vi "RealTimeAcq.vi"(4 "Frames/s":sgl=2.0, 5 "return to start":bool, 6 "Scan Axis":i8=3, 7 "Motion Board ID":T2=1 min=1 max=32 step=1, 8 "BKPT Shift":i32=75, 9 "stop out":bool) -> (0 "error out":errorcluster, 2 "Bd ID Out":T1)   [LabVIEW 2022 SP3]
uses:
  ScanningControl/Motion Controllers/-MotionRoutines/MotionGlobals.vi
  <instrlib>/Acqiris Dx/Acqiris Dx.lvlib
  <vilib>/Motion/FlexMotion/FunctionsVIs/Trajectory.llb/Load Acceleration/Deceleration.flx
  <vilib>/Motion/FlexMotion/CustomControls/CustomControls.llb/Axis To Control.flx
  <vilib>/Motion/FlexMotion/CustomControls/CustomControls.llb/Program.flx
  <instrlib>/Newport ESP301/Newport ESP301.lvlib
  <instrlib>/niScope/Acquire/Fetch/niScope Multi Fetch Binary 8.vi
  ScanningControl/-ScanSystem/DataHandling/ReverseDataI8.vi
  <vilib>/DAQmx/write.llb/DAQmx Write (Digital 1D Bool NChan 1Samp 1Line).vi
  <instrlib>/LeCroy Wave Series/LeCroy Wave Series.lvlib
  <vilib>/Motion/FlexMotion/FunctionsVIs/Trajectory.llb/Wait for Move Complete (8 axes).flx
panel:
  out "Frames":i32
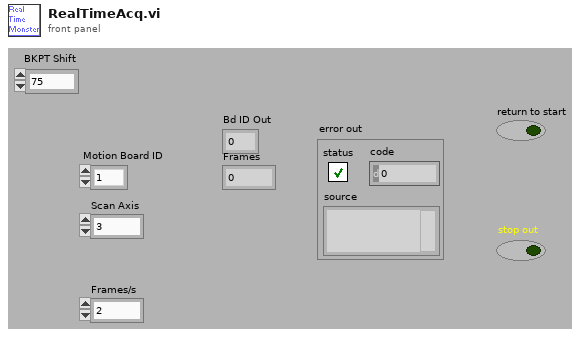
[diagram p1: front panel]
types:
  T1 = typedef "Bd Id Out" = u8
  T2 = typedef "Board Id" = u8
  T3 = cluster{"Time Step (ms)":i64, "Burst Ct":i8[], "Voltage Steps":sgl[], "Tabor Step Through?":bool}
  T4 = typedef "location.ctl" = enum16{"Automatic", "WCM Main", "Hawaii", "Columbia MM3000", "Columbia  NI System", "NYU", "RRI 2", "UHI Allen", "CUMC RT", "Chiba", "Stony Brook", "WCM Microscopy", "WCM Aeoretch", "WCM Optics Lab", "WCM Main 2Axis", "WCM Rotation", "WCM SAM SMAC", "SERI GP"}
  T5 = typedef "Program.flx" = u8
  T6 = cluster{"gain":dbl, bool, "Array":i16[][], "gain 2":dbl}
  T7 = typedef "Resource Out (Enum).flx" = u16
  T8 = typedef "Axis To Control.flx" = u16
  T9 = cluster{"returnedSamplesPerSeg":i32, "indexFirstPoint":i32, "sampTime":dbl, "vGain":dbl, "vOffset":dbl, "returnedSegments":i32, "nbrAvgWforms":i32, "actualTriggersInAcqLo":u32, "actualTriggersInAcqHi":u32, "reserved3":dbl, "actualDataSize":u32, "missingValue":dbl}
  T10 = cluster{"actualSamples":i32, "absoluteInitialX":dbl, "relativeInitialX":dbl, "xIncrement":dbl, "offset":dbl, "gain":dbl, "reserved1":dbl, "reserved2":dbl}[]
  T11 = cluster{"actualSamples":i32, "absoluteInitialX":dbl, "relativeInitialX":dbl, "xIncrement":dbl, "offset":dbl, "gain":dbl, "reserved1":dbl, "reserved2":dbl}
  T12 = cluster{"gain":dbl, bool, "Array":i16[][], "gain 2 Ch":dbl}
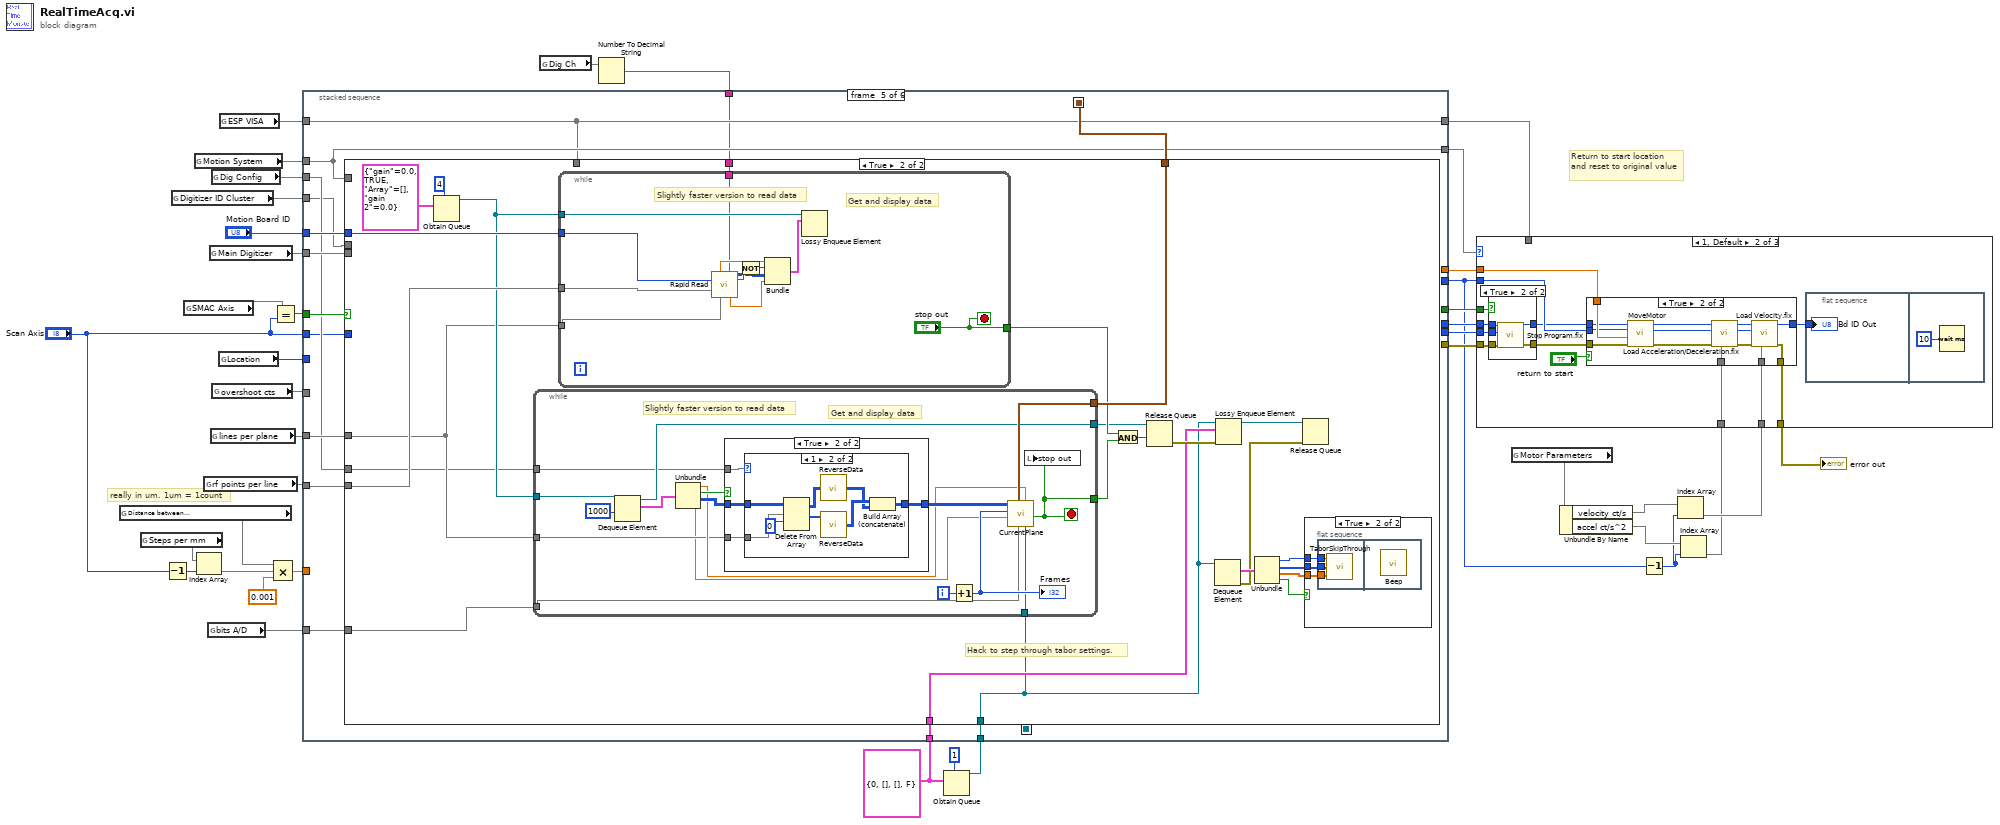
[diagram p0: block diagram]
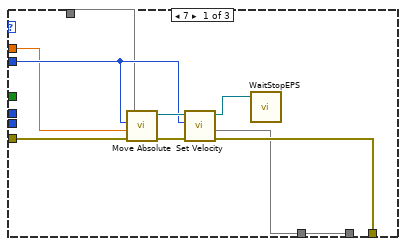
[diagram p2: hidden frame]
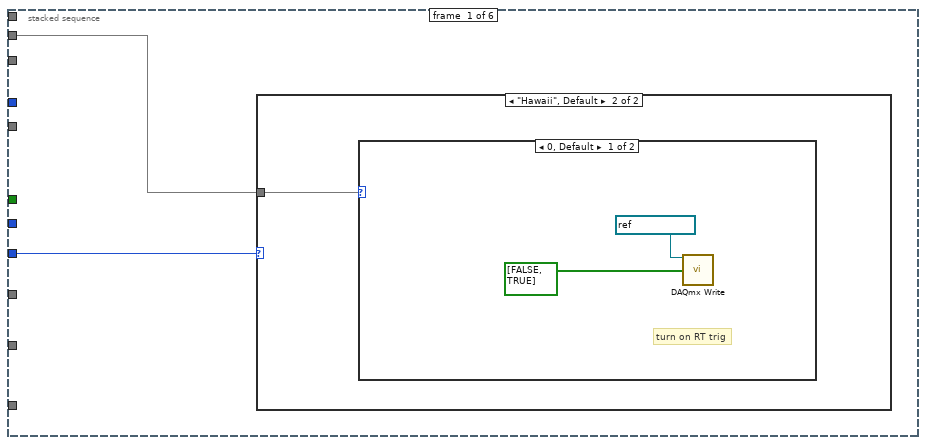
[diagram p6: hidden frame]
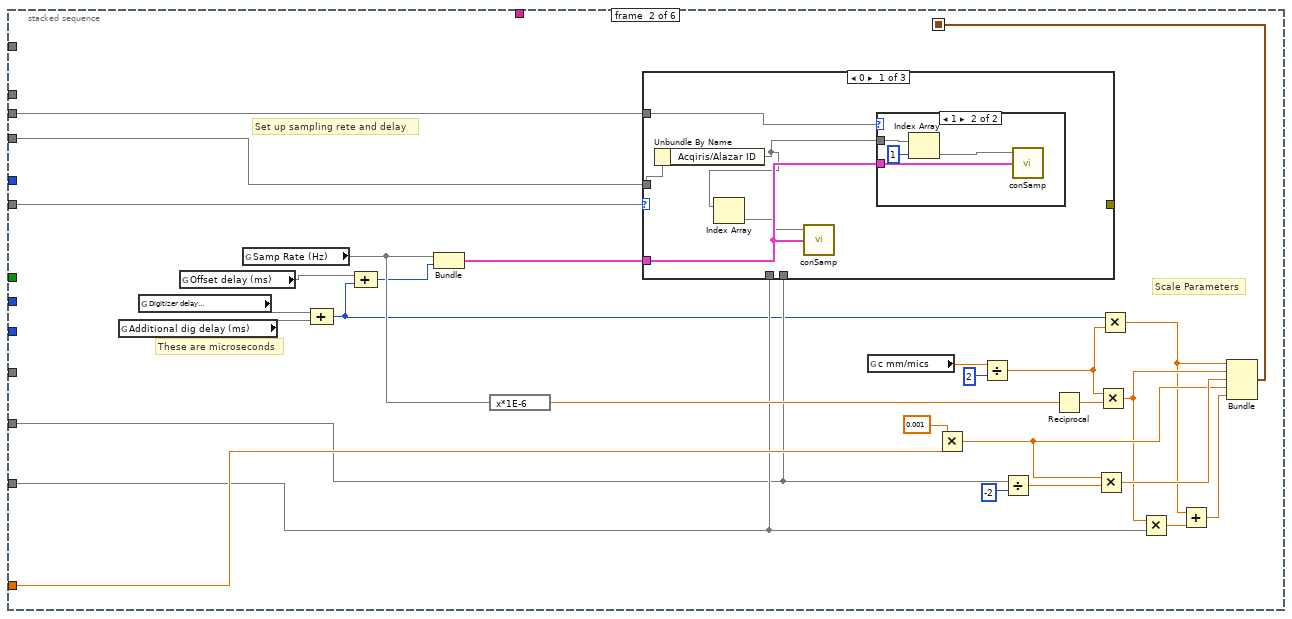
[diagram p9: hidden frame]
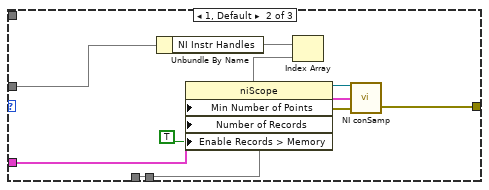
[diagram p11: hidden frame]
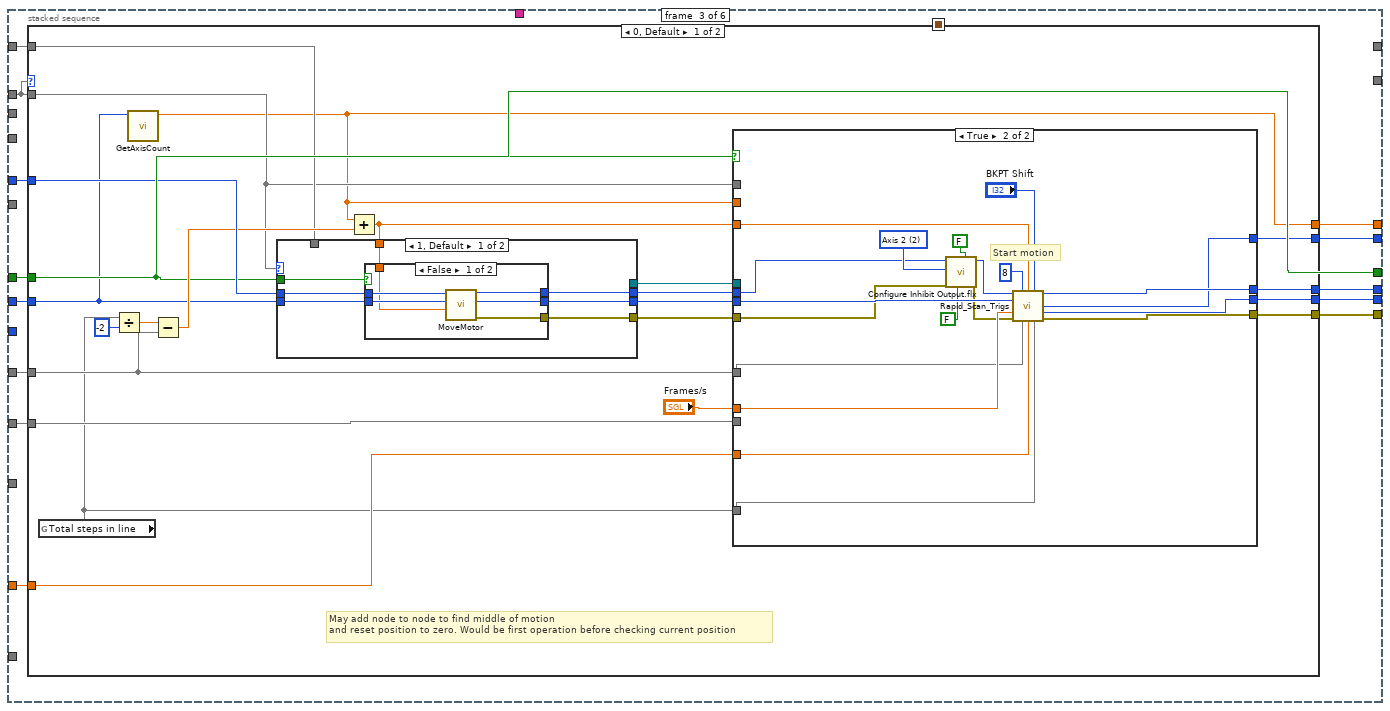
[diagram p13: hidden frame]
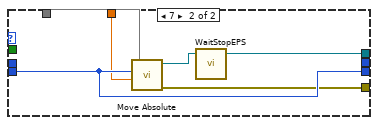
[diagram p15: hidden frame]
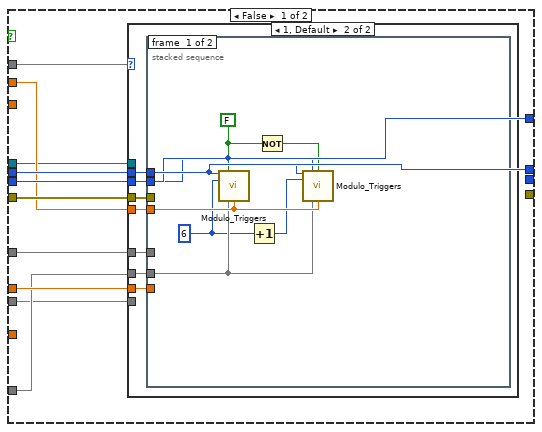
[diagram p16: hidden frame]
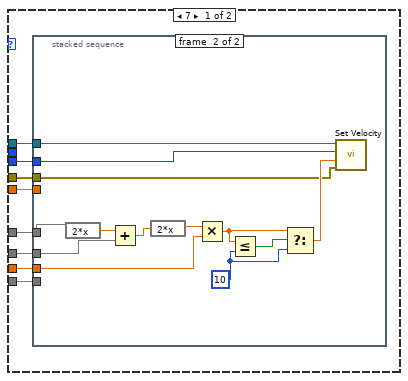
[diagram p17: hidden frame]
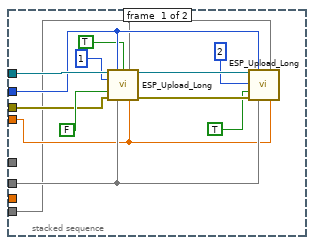
[diagram p18: hidden frame]
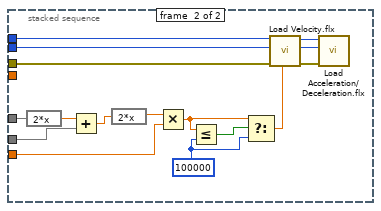
[diagram p19: hidden frame]
diagram:
  w11 = T3 {"Time Step (ms)"=0, "Burst Ct"=[], "Voltage Steps"=[], "Tabor Step Through?"=FALSE} ("Tabor")
  # "really in um. 1um = 1count"
  # "Return to start location and reset to original value"
  n1 = global read "MotionGlobals.vi" "Distance between\nscan lines (mm)"() -> (w29)
  n2 = global read "MotionGlobals.vi" "Steps per mm"() -> (w16)
  n3 = Decrement(x="Scan Axis") -> (x-1=w15:i8)
  n4 = global read "MotionGlobals.vi" "Digitizer ID Cluster"() -> (w9)
  n5 = global read "MotionGlobals.vi" "SMAC Axis"() -> (w13)
  n6 = global read "MotionGlobals.vi" "Motion System"() -> (w26)
  n7 = Index Array(array=w16, index=w15) -> (element=w14)
  n8 = global read "MotionGlobals.vi" "rf points per line"() -> (w39)
  n9 = global read "MotionGlobals.vi" "bits A/D"() -> (w17)
  n10 = global read "MotionGlobals.vi" "Main Digitizer"() -> (w27)
  n11 = global read "MotionGlobals.vi" "lines per plane"() -> (w40)
  n12 = global read "MotionGlobals.vi" "Dig Config"() -> (w20)
  n13 = global read "MotionGlobals.vi" "overshoot cts"() -> (w38)
  n14 = global read "MotionGlobals.vi" "Location"() -> (w21:T4)
  n15 = global read "MotionGlobals.vi" "ESP VISA"() -> (w25)
  n16 = Equal?(x=w13, y="Scan Axis") -> (x = y?=w31:bool)
  n17 = Compound Arithmetic op=MULTIPLY(w29, w14, 0.001) -> (w28:dbl)
  n18 = global read "MotionGlobals.vi" "Dig Ch"() -> (w19)
  n19 = Number To Decimal String(number=w19) -> (decimal integer string=w18:string)  [unwired: 1 in]
  n20 = Obtain Queue(max queue size (-1, unlimited)=1, element data type=w11) -> (queue out=w10:refnum<queue>)  [unwired: 3 in, 2 out]
  n21 = stacked-sequence {
    seq-local: [_ w63 _ _ _ _] -> [_ _ _ _ w286 _]
    seq-local: [_ _ _ w244 _ _] -> [_ _ _ _ _ w544]
    tunnel: w40 -> [_ w51 w98 _ w289 _]
    tunnel: [_ _ w105 _ _ _] -> w35
    tunnel: [_ _ w104 _ _ _] -> w37
    tunnel: w39 -> [_ w52 _ _ w288 _]
    tunnel: [_ _ w103 _ _ _] -> w36
    tunnel: [_ _ w94 _ _ _] -> w34
    tunnel: w38 -> [_ _ w101 _ _ _]
    tunnel: [_ _ w102 _ _ _] -> w1
    tunnel: "Motion Board ID" -> [_ _ w100 w245 w287 _]
    tunnel: [_ _ w95 _ _ _] -> w32
    tunnel: w31 -> [_ _ w95 _ w285 _]
    tunnel: "Scan Axis" -> [_ _ w96 w246 w278 _]
    tunnel: w28 -> [_ w56 w99 _ _ _]
    tunnel: w27 -> [_ w55 _ _ w284 _]
    tunnel: w26 -> [_ _ w93 w248 w283 _]
    tunnel: w25 -> [_ _ w97 _ w282 _]
    tunnel: [_ _ _ _ w283 _] -> w24
    tunnel: [_ _ _ _ w282 _] -> w23
    tunnel: w21 -> [w42 _ _ _ _ w547]
    tunnel: w20 -> [w41 w47 _ w247 w281 w545]
    tunnel: w18 -> [_ _ _ _ w280 _]
    tunnel: w17 -> [_ _ _ _ w279 _]
    tunnel: w11 -> [_ _ _ _ w277 _]
    tunnel: w10 -> [_ _ _ _ w276 _]
    tunnel: w9 -> [_ w46 _ _ w275 _]
    frame #0 {
      n22 = case shown="\"Hawaii\", Default" w42 {
        tunnel: w41 -> [_ w43]
        frame "UHI Allen", "CUMC RT" {
        }
        frame "Hawaii", Default {
          n23 = case shown="0, Default" w43 {
            frame 0, Default {
              # "turn on RT trig"
              n24 = call-poly <vilib>:"DAQmx Write.vi"("task/channels in"=refnum<k21> "DIO-L2 L3", "data"=bool[] [FALSE, TRUE]) -> ()  [unwired: 11 in, 3 out]
            }
            frame 44 {
            }
          }
        }
      }
    }
    frame #1 {
      # "Scale Parameters"
      # "Set up sampling rete and delay"
      # "These are microseconds"
      n25 = global read "MotionGlobals.vi" "Additional dig delay (ms)"() -> (w73)
      n26 = global read "MotionGlobals.vi" "Digitizer delay\n (ms)"() -> (w70)
      n27 = global read "MotionGlobals.vi" "Offset delay (ms)"() -> (w50)
      n28 = global read "MotionGlobals.vi" "Samp Rate (Hz)"() -> (w54)
      n29 = Compound Arithmetic op=ADD(w70, w73) -> (w49:i32)
      n30 = Compound Arithmetic op=ADD(w50, w49) -> (w48:i32)
      n31 = Bundle("Samp Rate (Hz)"=w54, w48) -> (w72:cluster{"Samp Rate (Hz)":void, i32})  [unwired: 1 out]
      n32 = expression code="x*1E-6"(w54) -> (w53:dbl)
      n33 = case shown="0" w55 {
        tunnel: w72 -> [w78 w88 _]
        tunnel: w46 -> [w76 w85 _]
        tunnel: w52 -> [_ w91 _]
        tunnel: w51 -> [_ w92 _]
        tunnel: [_ w87 _] -> _
        tunnel: w47 -> [w77 _ _]
        frame 0 {
          n34 = Unbundle By Name(w76) -> ("Acqiris/Alazar ID"=w75)
          n35 = Index Array(array=w75) -> (element=w74)  [unwired: 1 in]
          n36 = call "conSamp.vi"("Sampling"=w78, "InstrumentID"=w74) -> ()  [unwired: 1 in, 2 out]
          n37 = case shown="1" w77 {
            tunnel: w78 -> [_ w82]
            tunnel: w75 -> [_ w80]
            frame 0, Default {
            }
            frame 1 {
              n38 = Index Array(array=w80, index=1) -> (element=w79)
              n39 = call "conSamp.vi"("Sampling"=w82, "InstrumentID"=w79) -> ()  [unwired: 1 in, 2 out]
            }
          }
        }
        frame 1, Default {
          n40 = Unbundle By Name(w85) -> ("NI Instr Handles"=w84)
          n41 = Index Array(array=w84) -> (element=w83)  [unwired: 1 in]
          n42 = property class="niScope"(reference=w83, "Min Number of Points"=w91, "Number of Records"=w92, "Enable Records > Memory"=TRUE) -> (reference out=w90:refnum<k15>, error out=w89:errorcluster)  [unwired: 1 in]
          n43 = call "NI conSamp.vi"("error in"=w89, "Sampling"=w88, "InstrumentID"=w90) -> ("error out"=w87:errorcluster)  [unwired: 1 out]
        }
        frame 2 {
        }
      }
      n44 = global read "MotionGlobals.vi" "c mm/mics"() -> (w71:sgl)
      n45 = Multiply(x=0.001, y=w56) -> (x*y=w61:dbl)
      n46 = Divide(x=w71, y=2) -> (x/y=w64:sgl)
      n47 = Divide(x=w51, y=-2) -> (x/y=w66:dbl)
      n48 = Reciprocal(x=w53) -> (1/x=w69:dbl)
      n49 = Multiply(x=w61, y=w66) -> (x*y=w62:dbl)
      n50 = Multiply(x=w64, y=w69) -> (x*y=w60:dbl)
      n51 = Multiply(x=w49, y=w64) -> (x*y=w58:sgl)
      n52 = Multiply(x=w60, y=w52) -> (x*y=w59:dbl)
      n53 = Add(x=w58, y=w59) -> (x+y=w57:sgl)
      n54 = Bundle(w58, w60, w62, w61, w57) -> (w63:cluster{sgl, dbl, dbl, dbl, sgl})  [unwired: 1 out]
    }
    frame #2 {
      n55 = case shown="0, Default" w93 {
        tunnel: [w127 _] -> w105
        tunnel: [w126 _] -> w104
        tunnel: [w124 _] -> w103
        tunnel: [w123 _] -> w102
        tunnel: w101 -> [w121 _]
        tunnel: w100 -> [w117 _]
        tunnel: w99 -> [w116 _]
        tunnel: w98 -> [w114 _]
        tunnel: w97 -> [w113 _]
        tunnel: w96 -> [w107 _]
        tunnel: w95 -> [w110 _]
        tunnel: [w106 _] -> w94
        tunnel: w93 -> [w109 _]
        frame 0, Default {
          # "May add node to node to find middle of motion\nand reset position to zero. Would be first operation before checking current position"
          n56 = global read "MotionGlobals.vi" "Total steps in line"() -> (w108)
          n57 = Divide(x=w108, y=-2) -> (x/y=w122:dbl)
          n58 = call "GetAxisCount.vi"("Scan Axis"=w107) -> ("Counts"=w106:dbl)  [unwired: 10 in]
          n59 = Subtract(x=w122, y=w121) -> (x-y=w115:dbl)
          n60 = Add(x=w106, y=w115) -> (x+y=w111:dbl)
          n61 = case shown="1, Default" w109 {
            tunnel: [w133 _] -> w120
            tunnel: [w132 w149] -> w119
            tunnel: [w131 w146] -> w118
            tunnel: w117 -> [w135 _]
            tunnel: w107 -> [w134 w149]
            tunnel: w113 -> [_ w145]
            tunnel: [_ w147] -> w112
            tunnel: w111 -> [w130 w144]
            tunnel: w110 -> [w129 _]
            frame 1, Default {
              n62 = case shown="False" w129 {
                tunnel: w135 -> [w141 w143]
                tunnel: w134 -> [w140 w142]
                tunnel: [w139 w143] -> w133
                tunnel: [w138 w142] -> w132
                tunnel: [w137 _] -> w131
                tunnel: w130 -> [w136 _]
                frame False {
                  n63 = call "MoveMotor.vi"("Target Position (0)"=w136, "Axis or Vector Space"=w140, "Motion Bd ID"=w141) -> ("error out"=w137:errorcluster, "Resource Output"=w138:u16, "Bd ID Out"=w139:u8)  [unwired: 2 in, 4 out]
                }
                frame True {
                }
              }
            }
            frame 7 {
              n64 = call <instrlib>:"Move Absolute.vi"("Position (0 units)"=w144, "Axis (1)"=w149, "VISA resource name"=w145) -> ("error out"=w146:errorcluster, "VISA resource name out"=w148:refnum<visa-resource-name>)  [unwired: 3 in]
              n65 = call "WaitStopEPS.vi"("VISA resource name"=w148) -> ("VISA resource name out"=w147:refnum<visa-resource-name>)  [unwired: 2 in, 2 out]
            }
          }
          n66 = case shown="True" w110 {
            tunnel: "Frames/s" -> [w156 w243]
            tunnel: [_ w242] -> w127
            tunnel: [w159 w241] -> w126
            tunnel: [_ w240] -> w124
            tunnel: [w158 w239] -> w123
            tunnel: w108 -> [w153 w238]
            tunnel: w116 -> [_ w237]
            tunnel: w121 -> [w157 w236]
            tunnel: w120 -> [w159 w226]
            tunnel: w119 -> [w158 w235]
            tunnel: w118 -> [w155 w225]
            tunnel: w111 -> [_ w234]
            tunnel: w106 -> [w154 _]
            tunnel: w114 -> [w152 _]
            tunnel: w109 -> [w151 _]
            tunnel: w112 -> [w150 _]
            frame False {
              n67 = case shown="1, Default" w151 {
                tunnel: w153 -> [w167 w200]
                tunnel: w159 -> [_ w199]
                tunnel: w158 -> [w162 w198]
                tunnel: w157 -> [w164 w197]
                tunnel: w156 -> [w163 w196]
                tunnel: w155 -> [w160 w195]
                tunnel: w154 -> [w165 w194]
                tunnel: w152 -> [w166 _]
                tunnel: w150 -> [w161 _]
                frame 7 {
                  n68 = stacked-sequence {
                    tunnel: w167 -> [w172 w186]
                    tunnel: w166 -> [w169 _]
                    tunnel: w165 -> [w171 _]
                    tunnel: w164 -> [_ w187]
                    tunnel: w163 -> [_ w185]
                    tunnel: w162 -> [w170 w183]
                    tunnel: w161 -> [w180 w182]
                    tunnel: w160 -> [w175 w181]
                    frame #0 {
                      n69 = call "ESP_Upload_Long.vi"("Motion Settings In"=w180, "Axis"=w170, "Purge?"=TRUE, "lines per scan"=w169, "Program#"=1, "Reverse ?"=FALSE, "error in"=w175, 12:w172, "Offset"=w171) -> ("VISA resource name out"=w179:refnum<visa-resource-name>, "error out"=w174:errorcluster)  [unwired: 5 in]
                      n70 = call "ESP_Upload_Long.vi"("Motion Settings In"=w179, "Axis"=w170, "lines per scan"=w169, "Program#"=2, "Reverse ?"=TRUE, "error in"=w174, 12:w172, "Offset"=w171) -> ()  [unwired: 6 in, 2 out]
                    }
                    frame #1 {
                      w192 = 10
                      n71 = expression code="2*x"(w187) -> (w190:dbl)
                      n72 = Add(x=w190, y=w186) -> (x+y=w188:dbl)
                      n73 = expression code="2*x"(w188) -> (w189:dbl)
                      n74 = Multiply(x=w189, y=w185) -> (x*y=w193:sgl)
                      n75 = Less Or Equal?(x=w193, y=w192) -> (x <= y?=w191:bool)
                      n76 = Select(t=w193, s=w191, f=w192) -> (s? t:f=w184:sgl)
                      n77 = call <instrlib>:"Set Velocity.vi"("error in (no error)"=w181, "Velocity (units/s)"=w184, "Axis (1)"=w183, "VISA resource name"=w182) -> ()  [unwired: 2 in, 2 out]
                    }
                  }
                }
                frame 1, Default {
                  n78 = stacked-sequence {
                    tunnel: w194 -> [w208 _]
                    tunnel: w200 -> [w207 w221]
                    tunnel: w199 -> [w203 w217]
                    tunnel: w198 -> [w202 w216]
                    tunnel: w197 -> [_ w214]
                    tunnel: w196 -> [_ w212]
                    tunnel: w195 -> [_ w218]
                    frame #0 {
                      w201 = T5 6 ("Program (1)")
                      w206 = FALSE
                      n79 = call "Modulo_Triggers.vi"("Motion Settings In"=w203, "Axis"=w202, "Reverse ?"=w206, "Program (1)"=w201, 12:w207, "Offset"=w208) -> ()  [unwired: 2 in, 8 out]
                      n80 = Increment(x=w201) -> (x+1=w204:T5)
                      n81 = Not(x=w206) -> (.not. x?=w205:bool)
                      n82 = call "Modulo_Triggers.vi"("Motion Settings In"=w203, "Axis"=w202, "Reverse ?"=w205, "Program (1)"=w204, 12:w207, "Offset"=w208) -> ()  [unwired: 2 in, 8 out]
                    }
                    frame #1 {
                      w223 = 100000
                      n83 = expression code="2*x"(w214) -> (w213:dbl)
                      n84 = Add(x=w213, y=w221) -> (x+y=w210:dbl)
                      n85 = expression code="2*x"(w210) -> (w211:dbl)
                      n86 = Multiply(x=w211, y=w212) -> (x*y=w224:sgl)
                      n87 = Less Or Equal?(x=w224, y=w223) -> (x <= y?=w222:bool)
                      n88 = Select(t=w224, s=w222, f=w223) -> (s? t:f=w209:sgl)
                      n89 = call <vilib>:"Load Velocity.flx"("Velocity (10000)"=w209, "error in (no error)"=w218, "Axis or Vector Space"=w216, "Board ID"=w217) -> ("error out"=w219:errorcluster, "Resource Output"=w215:T7, "Bd ID Out"=w220:T1)  [unwired: 3 out]
                      n90 = call "Load Acceleration/Deceleration.flx"("error in (no error)"=w219, "Axis or Vector Space"=w215, "Board ID"=w220) -> ()  [unwired: 2 in, 5 out]
                    }
                  }
                }
              }
            }
            frame True {
              w229 = T8 2 items=["Axis 1"=1, "Axis 2"=2, "Axis 3"=3, "Axis 4"=4, "Axis 5"=5, "Axis 6"=6, "Axis 7"=7, "Axis 8"=8] ("Axis")
              # "Start motion"
              n91 = call <vilib>:"Configure Inhibit Output.flx"("Enable"=FALSE, "Polarity (Active Low)"=FALSE, "error in (no error)"=w225, "Axis"=w229, "Board ID"=w226) -> ("error out"=w232:errorcluster, "Bd ID Out"=w233:T1)  [unwired: 1 in, 4 out]
              n92 = call "Rapid_Scan_Trigs.vi"("Board ID"=w233, "Program (1)"=T5 8, "Start Position"=w234, "BKPT Shift"="BKPT Shift", "Scan Axis"=w235, "# frames/ s"=w243, "error in (no error)"=w232, "overshoot"=w236, "step interval"=w237, "Total Steps (one way)"=w238) -> ("Bd ID Out"=w241:u8, "Axis Resource out"=w239:u16, "Program ID"=w240:u8, "error out"=w242:errorcluster)  [unwired: 1 in, 1 out]
            }
          }
        }
        frame 8 {
        }
      }
    }
    frame #3 {
      n93 = case shown="4" w247 {
        tunnel: [_ w257] -> w244
        tunnel: w246 -> [_ w260]
        tunnel: w245 -> [_ w253]
        frame 0, Default {
        }
        frame 4 {
          n94 = global read "MotionGlobals.vi" "Switch T/R"() -> (w261)
          n95 = Decrement(x=w261) -> (x-1=w252:dbl)
          n96 = Replace Array Subset(array=bool[] [FALSE, FALSE, FALSE, FALSE, FALSE] ("XMIT"), new element=TRUE ("new element/subarray"), index=w252) -> (w249:bool[])
          n97 = call "5ChPulserTrigsNew.vi"("Motion Settings"=w253, "XMIT"=w249, "Axis"=w260) -> ("5CH Pulser Tasks"=w259:refnum<k21>[])  [unwired: 6 in, 1 out]
          n98 = for {
            tunnel: w259 -> [w273] mode=indexing
            tunnel: [w272] -> w257 mode=indexing
            tunnel: [w271] -> w256
            n99 = call <vilib>:"DAQmx Start Task.vi"("task/channels in"=w273) -> ("task out"=w272:refnum<k21>, "error out"=w271:errorcluster)  [unwired: 1 in, 12 out]
          }
          n100 = for {
            tunnel: bool[][] [[TRUE], [FALSE]] ("data") -> [w265] mode=indexing
            tunnel: w256 -> [_]
            tunnel: [w264] -> w254
            n101 = flat-sequence {
              tunnel: w265 -> [w268]
              tunnel: [w268] -> w266
              tunnel: w266 -> [w270]
              tunnel: [w269] -> w264
              frame #0 {
                n102 = Wait (ms)(milliseconds to wait=u32 25) -> ()  [unwired: 1 out]
              }
              frame #1 {
                n103 = call "DAQ Assistant"("data"=w270) -> ("error out"=w269:errorcluster)  [unwired: 17 in, 1 out]
              }
            }
          }
          n104 = for {
            N: 3 -> [_]
            tunnel: w253 -> [w263]
            tunnel: w254 -> [w262]
            n105 = call "ForceBreakPt.vi"("error in"=w262, "Bd ID in"=w263) -> ()  [unwired: 2 out]
          }
        }
      }
      n106 = case shown="0, Default" w248 {
        tunnel: w245 -> [w274 _]
        frame 0, Default {
          n107 = call "CheckLimStat.vi"("Motion Board ID"=w274) -> ()
        }
        frame 1, 7, 8 {
        }
      }
    }
    frame #4 {
      n108 = case shown="True" w285 {
        tunnel: w289 -> [w303 w476]
        tunnel: w288 -> [w304 w493]
        tunnel: w287 -> [w301 w492]
        tunnel: w286 -> [w300 w490]
        tunnel: w284 -> [w299 _]
        tunnel: w283 -> [w298 _]
        tunnel: w282 -> [w297 _]
        tunnel: w281 -> [_ w475]
        tunnel: w280 -> [w296 w473]
        tunnel: w279 -> [w295 w472]
        tunnel: w278 -> [w293 _]
        tunnel: w277 -> [_ w471]
        tunnel: w276 -> [w292 w470]
        tunnel: w275 -> [w290 _]
        frame False {
          n109 = global read "MotionGlobals.vi" "DigTimeOut"() -> (w294)
          n110 = while {
            tunnel: w304 -> [w332]
            tunnel: w303 -> [w323]
            shift-right: [w331] -> _
            shift-left: TRUE -> [w316]
            tunnel: w301 -> [w330]
            tunnel: w300 -> [w326]
            tunnel: w299 -> [w324]
            tunnel: w298 -> [w317]
            tunnel: w297 -> [w318]
            tunnel: w296 -> [w311]
            tunnel: w295 -> [w309]
            tunnel: w294 -> [w308]
            tunnel: w293 -> [w307]
            tunnel: w292 -> [w306]
            tunnel: [w306] -> w291
            tunnel: w290 -> [w305]
            i -> [w325]
            stop <- w329 stop-if-true
            # "Display data"
            # "Get data"
            # "This is slower version for heavier mass motors. Scan stop, read data, scan etc"
            n111 = Select(t="1", s=w316, f="2") -> (s? t:f=w313:string)
            n112 = Select(t=T5 6 ("Program (1)"), s=w316, f=T5 7 ("Program (1)")) -> (s? t:f=w321:T5)
            n113 = case shown="1, Default" w324 {
              tunnel: w332 -> [w352 w397 _]
              tunnel: w323 -> [w351 w392 w431]
              tunnel: w330 -> [w364 w410 w421]
              tunnel: [w363 w409 w445] -> w328
              tunnel: w321 -> [w359 w408 w444]
              tunnel: [w345 w402 w427] -> w310
              tunnel: w305 -> [w338 w385 w419]
              tunnel: w316 -> [w348 w399 w426]
              tunnel: [w349 w400 w428] -> w322
              tunnel: w317 -> [w343 _ w439]
              tunnel: w318 -> [w347 _ w442]
              tunnel: w313 -> [w346 _ w441]
              tunnel: [w341 w389 w425] -> w312
              tunnel: w311 -> [_ w398 _]
              tunnel: w308 -> [w340 w386 w430]
              tunnel: w307 -> [_ _ w420]
              frame 0 {
                n114 = Unbundle By Name(w338) -> ("Acqiris/Alazar ID"=w337)
                n115 = Index Array(array=w337) -> (element=w336)  [unwired: 1 in]
                n116 = call <instrlib>:"Configure Memory Settings.vi"("Number of Samples (1000)"=w352, "Number of Segments (1)"=w351, "Instrument ID"=w336) -> ("error out"=w362:errorcluster, "dup Instrument ID"=w360:u32)  [unwired: 1 in, 2 out]
                n117 = call <instrlib>:"Start Acquisition.vi"("error in (no error)"=w362, "Instrument ID"=w360) -> ("error out"=w358:errorcluster, "dup Instrument ID"=w361:u32)  [unwired: 2 in]
                n118 = stacked-sequence {
                  tunnel: w358 -> [w382]
                  tunnel: [w382] -> w357
                  frame #0 {
                    n119 = Wait (ms)(milliseconds to wait=20) -> ()  [unwired: 1 out]
                  }
                }
                n120 = case shown="7" w343 {
                  tunnel: w364 -> [w370 _]
                  tunnel: [w369 _] -> w363
                  tunnel: w359 -> [w368 _]
                  tunnel: w357 -> [w367 w375]
                  tunnel: [w366 w372] -> w356
                  tunnel: w347 -> [_ w374]
                  tunnel: w346 -> [_ w373]
                  tunnel: [_ w371] -> w344
                  frame 0, Default {
                    n121 = call <vilib>:"Run Program.flx"("error in (no error)"=w367, "Program (1)"=w368, "Board ID"=w370) -> ("error out"=w366:errorcluster, "Bd ID Out"=w369:T1)  [unwired: 4 out]
                  }
                  frame 7 {
                    n122 = call <instrlib>:"Execute Program.vi"("error in (no error)"=w375, "Program Name"=w373, "VISA resource name"=w374) -> ("error out"=w372:errorcluster, "VISA resource name out"=w371:refnum<visa-resource-name>)  [unwired: 3 in]
                  }
                }
                n123 = expression code="x*1000"(w340) -> (w339:dbl)
                n124 = stacked-sequence {
                  tunnel: w356 -> [w379]
                  tunnel: [w379] -> w355
                  frame #0 {
                    n125 = Wait (ms)(milliseconds to wait=20) -> ()  [unwired: 1 out]
                  }
                }
                n126 = call "WaitForSegs.vi"("Acqiris ID"=w361, "lines per plane"=w351, "error in"=w355, "Timeout"=w339) -> ("dup Instrument ID"=w354:u32, "error out"=w353:errorcluster)  [unwired: 2 out]
                n127 = call "GetWaveform.vi"("Acq ID Out"=w354, "Num Samps"=w352, "Num Segs"=w351, "error in"=w353) -> ("Acquired Waveform16 bit"=w350:i16[][], "dataDesc"=w342:T9, "error out"=w345:errorcluster)  [unwired: 2 in, 7 out]
                n128 = case shown="True" w348 {
                  tunnel: w350 -> [w376 w378]
                  tunnel: [w376 w377] -> w349
                  frame False {
                  }
                  frame True {
                    n129 = call "ReverseData.vi"("Array in"=w378) -> ("Array out"=w377:i16[][])
                  }
                }
                n130 = Unbundle By Name(w342) -> ("vGain"=w341:dbl)
                n131 = case shown="7" w343 {
                  tunnel: w344 -> [_ w365]
                  frame 0, Default {
                  }
                  frame 7 {
                    n132 = call "WaitStopEPS.vi"("VISA resource name"=w365) -> ()  [unwired: 2 in, 3 out]
                  }
                }
              }
              frame 1, Default {
                n133 = Unbundle By Name(w385) -> ("NI Instr Handles"=w384)
                n134 = Index Array(array=w384) -> (element=w383)  [unwired: 1 in]
                n135 = property class="niScope"(reference=w383, "Number of Records"=w392, "Min Number of Points"=w397) -> (reference out=w404:refnum<k15>, error out=w403:errorcluster)  [unwired: 1 in]
                n136 = call <instrlib>:"niScope Initiate Acquisition.vi"("instrument handle"=w404, "error in"=w403) -> ("instrument handle out"=w396:refnum<k15>, "error out"=w407:errorcluster)  [unwired: 1 in, 11 out]
                n137 = stacked-sequence {
                  tunnel: w407 -> [w417]
                  tunnel: [w417] -> w406
                  frame #0 {
                    n138 = Wait (ms)(milliseconds to wait=u32 5) -> ()  [unwired: 1 out]
                  }
                }
                n139 = call <vilib>:"Run Program.flx"("error in (no error)"=w406, "Program (1)"=w408, "Board ID"=w410) -> ("error out"=w405:errorcluster, "Bd ID Out"=w409:T1)  [unwired: 4 out]
                n140 = stacked-sequence {
                  tunnel: w405 -> [w414]
                  tunnel: [w414] -> w394
                  frame #0 {
                    n141 = Wait (ms)(milliseconds to wait=u32 20) -> ()  [unwired: 1 out]
                  }
                }
                n142 = property class="niScope"(reference=w396, error in=w394, "Fetch Record Number"=0, "Fetch Number of Records"=-1) -> (reference out=w395:refnum<k15>, error out=w393:errorcluster)
                n143 = call-poly <instrlib>:"niScope Fetch (poly).vi"("timeout"=w386, "error in"=w393, "numSamples"=w397, "channels"=w398, "instrument handle"=w395) -> ("error out"=w402:errorcluster, "wfm"=w401:i8[][], "wfm info"=w391:T10)  [unwired: 4 out]
                n144 = case shown="True" w399 {
                  tunnel: w401 -> [w411 w413]
                  tunnel: [w411 w412] -> w400
                  frame False {
                  }
                  frame True {
                    n145 = call-poly "ReversePoly.vi"("Array in"=w413) -> ("Array out"=w412:i8[][])
                  }
                }
                n146 = Index Array(array=w391) -> (element=w390:T11)  [unwired: 1 in]
                n147 = Unbundle By Name(w390) -> ("gain"=w389:dbl)
              }
              frame 2 {
                w438 = FALSE ("Continuous Acquisition Mode (T: On)")
                w436 = u16 2 items=["RealTime", "RIS", "Sequence", "Roll", "WaveStream"] ("Sample Mode (0: RealTime)")
                n148 = Unbundle By Name(w419) -> ("LeCroy VISA"=w418)
                n149 = call <instrlib>:"Configure Continuous Acquisition.vi"("Auto Trigger Enabled (T: Normal)"=w438, "Continuous Acquisition Mode (T: On)"=w438, "VISA resource name"=w418) -> ("error out"=w435:errorcluster, "VISA resource name out"=w437:refnum<visa-resource-name>)  [unwired: 7 in]
                n150 = call <instrlib>:"Configure Sample Mode.vi"("error in (no error)"=w435, "Number of Segments (2)"=w431, "Sample Mode (0: RealTime)"=w436, "VISA resource name"=w437) -> ("error out"=w434:errorcluster, "VISA resource name out"=w432:refnum<visa-resource-name>)  [unwired: 6 in]
                n151 = call <instrlib>:"Initiate.vi"("error in (no error)"=w434, "VISA resource name"=w432) -> ("error out"=w433:errorcluster)  [unwired: 8 in, 1 out]
                n152 = case shown="0, Default" w439 {
                  tunnel: w421 -> [w451 _]
                  tunnel: [w450 _] -> w445
                  tunnel: w444 -> [w449 _]
                  tunnel: w433 -> [w448 w456]
                  tunnel: [w447 w453] -> w443
                  tunnel: w442 -> [_ w455]
                  tunnel: w441 -> [_ w454]
                  tunnel: [_ w452] -> w440
                  frame 0, Default {
                    n153 = call <vilib>:"Run Program.flx"("error in (no error)"=w448, "Program (1)"=w449, "Board ID"=w451) -> ("error out"=w447:errorcluster, "Bd ID Out"=w450:T1)  [unwired: 4 out]
                  }
                  frame 7 {
                    n154 = call <instrlib>:"Execute Program.vi"("error in (no error)"=w456, "Program Name"=w454, "VISA resource name"=w455) -> ("error out"=w453:errorcluster, "VISA resource name out"=w452:refnum<visa-resource-name>)  [unwired: 3 in]
                  }
                }
                n155 = expression code="x*1000"(w430) -> (w422:dbl)
                n156 = stacked-sequence {
                  tunnel: w443 -> [w457]
                  tunnel: [w457] -> w423
                  frame #0 {
                    n157 = Wait (ms)(milliseconds to wait=40) -> ()  [unwired: 1 out]
                  }
                }
                n158 = call-poly <vilib>:"Wait for Move Complete.flx"("Timeout (10000 ms)"=w422, "error in (no error)"=w423, "Axis or Vector Space"=w420, "Board ID"=w421) -> ("error out"=w424:errorcluster)  [unwired: 4 in, 3 out]
                n159 = call "GetAcqSeqLeCroy.vi"("errorin"=w424, "save?"=FALSE, "Reverse?"=w426) -> ("Raw VGain (scale)"=w425:dbl, "Data Array"=w428:i16[][], "error out"=w427:errorcluster)  [unwired: 18 in, 4 out]
                n160 = case shown="7" w439 {
                  tunnel: w440 -> [_ w446]
                  frame 0, Default {
                  }
                  frame 7 {
                    n161 = call "WaitStopEPS.vi"("VISA resource name"=w446) -> ()  [unwired: 2 in, 3 out]
                  }
                }
              }
            }
            n162 = case shown="No Error" w310 {
              selector: w310 -> [w463 w468]
              tunnel: [w464 w468] -> w327
              tunnel: [w467 TRUE] -> w329
              tunnel: w326 -> [w466 _]
              tunnel: w325 -> [w465 _]
              tunnel: w322 -> [w462 _]
              tunnel: w312 -> [w461 _]
              tunnel: w309 -> [w460 _]
              tunnel: w306 -> [w459 _]
              frame No Error {
                n163 = call "CurrentPlane.vi"("queue In"=w459, "gain"=w461, "bits A/D"=w460, "Axis Vals"=w466, "error in"=w463, "Frame"=w465, "Data"=w462) -> ("error out"=w464:errorcluster, "stop out"=w467:bool)  [unwired: 3 in]
              }
              frame Error {
              }
            }
            n164 = local write "Frames"(w325) -> ()
            n165 = case shown="1, Default" w317 {
              tunnel: w328 -> [_ w335]
              tunnel: w327 -> [_ w334]
              tunnel: w321 -> [_ w333]
              frame 7 {
              }
              frame 1, Default {
                n166 = call <vilib>:"Stop Program.flx"("error in (no error)"=w334, "Program (1)"=w333, "Board ID"=w335) -> ()  [unwired: 6 out]
              }
            }
            n167 = Not(x=w316) -> (.not. x?=w331:bool)
          }
          n168 = Release Queue(queue=w291) -> ()  [unwired: 2 in, 3 out]
        }
        frame True {
          # "Hack to step through tabor settings."
          n169 = Obtain Queue(max queue size (-1, unlimited)=4, element data type=T6 {"gain"=0.0, TRUE, "Array"=[], "gain 2"=0.0}) -> (queue out=w489:refnum<queue>)  [unwired: 2 in, 3 out]
          n170 = while {
            tunnel: w490 -> [w515]
            tunnel: w489 -> [w508]
            tunnel: [w511] -> w487
            tunnel: [w513] -> w486
            tunnel: w470 -> [w504]
            tunnel: w475 -> [w503]
            tunnel: w476 -> [w502]
            tunnel: w472 -> [w500]
            i -> [w516]
            stop <- w511 stop-if-true
            # "Slightly faster version to read data"
            # "Get and display data"
            n171 = Dequeue Element(queue=w508, timeout in ms (-1)=1000) -> (queue out=w513:refnum<queue>, element=w510:T6)  [unwired: 1 in, 2 out]
            n172 = Unbundle(w510) -> ("gain"=w505:dbl, w506:bool, "Array"=w507:i16[][], "gain 2"=w501:dbl)
            n173 = case shown="True" w506 {
              tunnel: w507 -> [w517 w521]
              tunnel: [w517 w520] -> w509
              tunnel: w503 -> [_ w519]
              tunnel: w502 -> [_ w518]
              frame False {
              }
              frame True {
                n174 = case shown="1" w519 {
                  tunnel: w521 -> [w523 w531]
                  tunnel: [w522 w525] -> w520
                  tunnel: w518 -> [_ w530]
                  frame 0, Default {
                    n175 = call "ReverseData.vi"("Array in"=w523) -> ("Array out"=w522:i16[][])
                  }
                  frame 1 {
                    n176 = Delete From Array(array=w531, length=w530, index (row)=0 ("disabled index (col)")) -> (deleted portion=w528:i16[], array with subset deleted=w529:i16[][])  [unwired: 1 in]
                    n177 = call "ReverseData.vi"("Array in"=w529) -> ("Array out"=w526:i16[][])
                    n178 = call "ReverseData.vi"("Array in"=w528) -> ("Array out"=w527:i16[][])
                    n179 = Build Array (concatenate)(w527, w526) -> (w525:i16[][])
                  }
                }
              }
            }
            n180 = Increment(x=w516) -> (x+1=w514:i32)
            "Frames" <- w514
            n181 = call "CurrentPlane.vi"("queue In"=w504, "gain"=w505, "bits A/D"=w500, "Axis Vals"=w515, "gain 2 Ch"=w501, "Frame"=w514, "Data"=w509) -> ("stop out"=w511:bool)  [unwired: 3 in, 1 out]
            n182 = local write "stop out"(w511) -> ()
          }
          n183 = while {
            tunnel: w476 -> [w541]
            tunnel: w493 -> [w542]
            tunnel: w492 -> [w543]
            tunnel: w489 -> [w540]
            tunnel: ["stop out"] -> w488
            tunnel: w473 -> [w533]
            stop <- "stop out" stop-if-true
            # "Slightly faster version to read data"
            # "Get and display data"
            n184 = call "Rapid Read.vi"(3:w533, "Motion Settings"=w543, "Location"=w542, "Pause?"=w541) -> ("gain"=w535:dbl, "Array"=w537:i16[][], "Reverse?"=w538:bool, "gain 2 Ch"=w534:dbl)  [unwired: 6 in, 2 out]
            n185 = Not(x=w538) -> (.not. x?=w532:bool)
            n186 = Bundle("gain"=w535, w532, "Array"=w537, "gain 2 Ch"=w534) -> (w536:T12)  [unwired: 1 out]
            n187 = Lossy Enqueue Element(queue=w540, element=w536) -> ()  [unwired: 1 in, 4 out]
          }
          n188 = And(x=w488, y=w487) -> (x .and. y?=w485:bool)
          n189 = Release Queue(queue=w486, force destroy? (F)=w485) -> (error out=w478:errorcluster)  [unwired: 1 in, 2 out]
          n190 = Dequeue Element(queue=w470) -> (element=w483:T3, error out=w474:errorcluster)  [unwired: 2 in, 2 out]
          n191 = Lossy Enqueue Element(queue=w470, element=w471, error in (no error)=w478) -> (queue out=w477:refnum<queue>)  [unwired: 3 out]
          n192 = Unbundle(w483) -> ("Time Step (ms)"=w481:i64, "Burst Ct"=w480:i8[], "Voltage Steps"=w479:sgl[], "Tabor Step Through?"=w482:bool)
          n193 = Release Queue(queue=w477, error in (no error)=w474) -> ()  [unwired: 1 in, 3 out]
          n194 = case shown="True" w482 {
            tunnel: w481 -> [_ w496]
            tunnel: w480 -> [_ w495]
            tunnel: w479 -> [_ w494]
            frame False {
            }
            frame True {
              n195 = flat-sequence {
                tunnel: w496 -> [w499]
                tunnel: w495 -> [w498]
                tunnel: w494 -> [w497]
                frame #0 {
                  n196 = call "TaborSkipThrough.vi"("Voltage Steps"=w497, "Burst Ct"=w498, "Time Step (ms)"=w499) -> ()  [unwired: 9 in]
                }
                frame #1 {
                  n197 = call <vilib>:"Beep.vi"() -> ()  [unwired: 12 in]
                }
              }
            }
          }
        }
      }
    }
    frame #5 {
      n198 = case shown="\"Hawaii\", Default" w547 {
        frame "Hawaii", Default {
          # "turn off real time trig"
          n199 = call-poly <vilib>:"DAQmx Write.vi"("task/channels in"=refnum<k21> "DIO-L2 L3", "data"=bool[] [TRUE, FALSE]) -> ()  [unwired: 11 in, 3 out]
        }
        frame "UHI Allen", "CUMC RT" {
        }
      }
      n200 = case shown="4, 5" w545 {
        tunnel: w544 -> [_ w548]
        frame 0, Default {
        }
        frame 4, 5 {
          n201 = for {
            tunnel: w548 -> [w551] mode=indexing
            n202 = call <vilib>:"DAQmx Stop Task.vi"("task/channels in"=w551) -> ("task out"=w550:refnum<k21>, "error out"=w549:errorcluster)  [unwired: 13 in]
            n203 = call <vilib>:"DAQmx Clear Task.vi"("task in"=w550, "error in"=w549) -> ()  [unwired: 13 in, 1 out]
          }
        }
      }
      n204 = local write "stop out"(FALSE ("stop out")) -> ()
    }
  }
  n205 = global read "MotionGlobals.vi" "Motor Parameters"() -> (w4)
  n206 = Unbundle By Name(w4) -> ("velocity ct/s"=w7, "accel ct/s^2"=w6)
  n207 = Decrement(x=w1) -> (x-1=w5:u16)
  n208 = Index Array(array=w7, index=w5) -> (element=w3)
  n209 = Index Array(array=w6, index=w5) -> (element=w2)
  n210 = case shown="1, Default" w24 {
    tunnel: w1 -> [w559 w575 _]
    tunnel: w37 -> [_ w574 _]
    tunnel: w36 -> [_ w573 _]
    tunnel: w35 -> [w556 w572 w601]
    tunnel: w34 -> [w558 w571 _]
    tunnel: w32 -> [_ w567 _]
    tunnel: w23 -> [w557 _ _]
    tunnel: [w555 w566 w601] -> w22
    tunnel: w3 -> [w554 w564 _]
    tunnel: w2 -> [_ w563 _]
    frame 7 {
      n211 = call <instrlib>:"Move Absolute.vi"("error in (no error)"=w556, "Position (0 units)"=w558, "Axis (1)"=w559, "VISA resource name"=w557) -> ("error out"=w562:errorcluster, "VISA resource name out"=w560:refnum<visa-resource-name>)  [unwired: 2 in]
      n212 = call <instrlib>:"Set Velocity.vi"("error in (no error)"=w562, "Velocity (units/s)"=w554, "Axis (1)"=w559, "VISA resource name"=w560) -> ("error out"=w555:errorcluster, "VISA resource name out"=w561:refnum<visa-resource-name>)  [unwired: 2 in]
      n213 = call "WaitStopEPS.vi"("VISA resource name"=w561) -> ()  [unwired: 2 in, 3 out]
    }
    frame 1, Default {
      n214 = case shown="True" w567 {
        tunnel: w574 -> [w595 w600]
        tunnel: w573 -> [_ w599]
        tunnel: w572 -> [w594 w598]
        tunnel: [w595 w597] -> w570
        tunnel: [w594 w596] -> w569
        frame False {
        }
        frame True {
          n215 = call <vilib>:"Stop Program.flx"("error in (no error)"=w598, "Program (1)"=w599, "Board ID"=w600) -> ("error out"=w596:errorcluster, "Bd ID Out"=w597:T1)  [unwired: 4 out]
        }
      }
      n216 = case shown="True" "return to start" {
        tunnel: w575 -> [_ w585]
        tunnel: w571 -> [_ w591]
        tunnel: w570 -> [w577 w584]
        tunnel: w569 -> [w576 w583]
        tunnel: [w577 w590] -> w568
        tunnel: [w576 w589] -> w566
        tunnel: w564 -> [_ w579]
        tunnel: w563 -> [_ w578]
        frame False {
        }
        frame True {
          n217 = call "MoveMotor.vi"("error in (no error)"=w583, "Target Position (0)"=w591, "Axis or Vector Space"=w585, "Motion Bd ID"=w584) -> ("error out"=w581:errorcluster, "Resource Output"=w580:u16, "Bd ID Out"=w582:u8)  [unwired: 1 in, 4 out]
          n218 = call "Load Acceleration/Deceleration.flx"("Acceleration (100000)"=w578, "error in (no error)"=w581, "Axis or Vector Space"=w580, "Board ID"=w582) -> ("error out"=w588:errorcluster, "Resource Output"=w586:T7, "Bd ID Out"=w587:T1)  [unwired: 1 in, 2 out]
          n219 = call <vilib>:"Load Velocity.flx"("Velocity (10000)"=w579, "error in (no error)"=w588, "Axis or Vector Space"=w586, "Board ID"=w587) -> ("error out"=w589:errorcluster, "Bd ID Out"=w590:T1)  [unwired: 4 out]
        }
      }
      n220 = flat-sequence {
        tunnel: w568 -> [w592]
        frame #0 {
          "Bd ID Out" <- w592
        }
        frame #1 {
          n221 = Wait (ms)(milliseconds to wait=u32 10) -> ()  [unwired: 1 out]
        }
      }
    }
    frame 8 {
    }
  }
  "error out" <- w22
